vi "DownloadDevMode.vi"(5 "LocalCompiledPath":path, 6 "error in":errorcluster, 9 "Downloader in":refnum<class "Downloader.lvclass">) -> (0 "error out":errorcluster, 2 "Path on Target":path, 3 "Downloader out":refnum<class "Downloader.lvclass">)   [LabVIEW 2014, in "Downloader.lvclass"]
uses:
  Downloader.lvclass
  Downloader.lvclass/Downloader.ctl
  MessageBox/MessageBox.lvclass
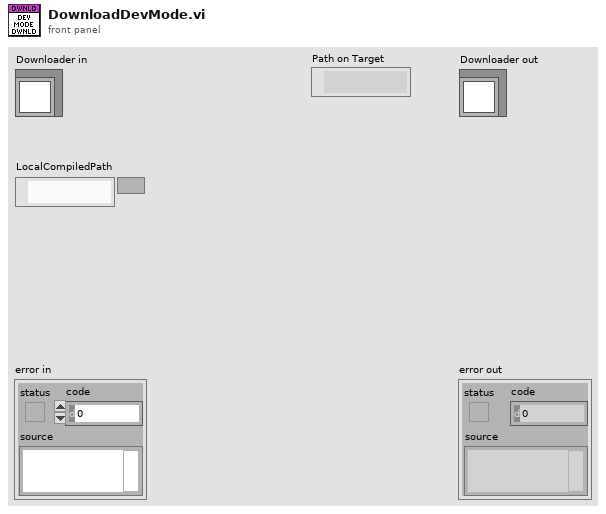
[diagram p1: front panel]
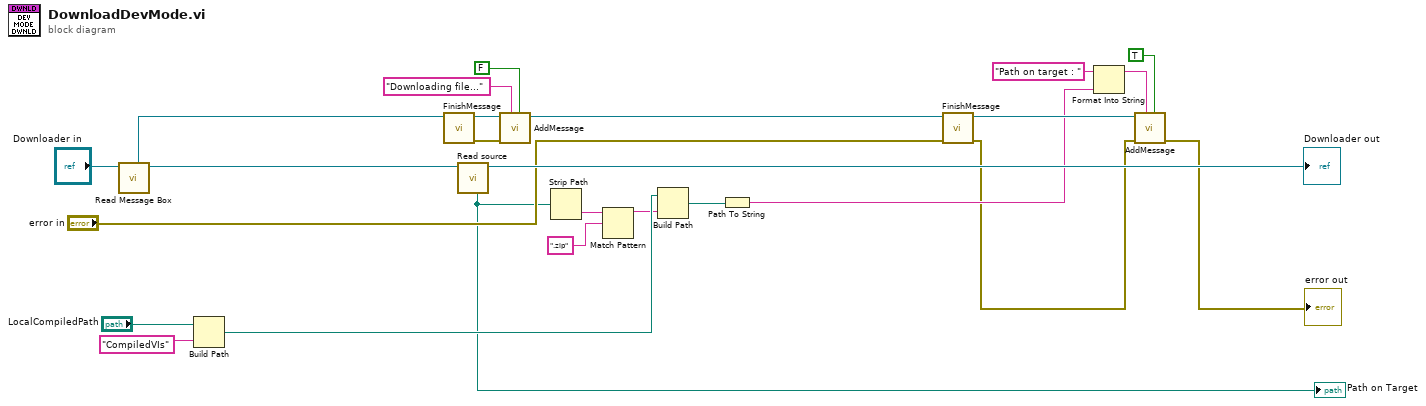
[diagram p0: block diagram]
diagram:
  n1 = call "Read Message Box.vi"("Downloader in"="Downloader in") -> ("Downloader out"=w13:refnum<class "Downloader.lvclass">, "Message Box"=w14:refnum<class "MessageBox.lvclass">)  [unwired: 7 in]
  n2 = Build Path(base path="LocalCompiledPath", name or relative path="CompiledVIs") -> (appended path=w7:path)
  n3 = call "FinishMessage.vi"("MessageBox in"=w14) -> ("error out"=w23:errorcluster, "MessageBox out"=w22:refnum<class "MessageBox.lvclass">)  [unwired: 7 in]
  n4 = call "Read source.vi"("Downloader in"=w13) -> ("Downloader out"=→"Downloader out":refnum<class "Downloader.lvclass">, "source"=w1:path)  [unwired: 7 in]
  "Path on Target" <- w1
  n5 = call "AddMessage.vi"("add newline"=FALSE, "message"="Downloading file...", "error in"=w23, "MessageBox in"=w22) -> ("MessageBox out"=w20:refnum<class "MessageBox.lvclass">)  [unwired: 4 in, 1 out]
  n6 = Strip Path(path=w1) -> (name=w4:string)  [unwired: 1 out]
  n7 = Match Pattern(string=w4, regular expression=".zip") -> (before substring=w2:string)  [unwired: 1 in, 3 out]
  n8 = Build Path(base path=w7, name or relative path=w2) -> (appended path=w5:path)
  n9 = Path To String(path=w5) -> (string=w9:string)
  n10 = call "FinishMessage.vi"("error in"="error in", "MessageBox in"=w20) -> ("error out"=w8:errorcluster, "MessageBox out"=w19:refnum<class "MessageBox.lvclass">)  [unwired: 6 in]
  n11 = Format Into String(initial string="Path on target : ", w9) -> (resulting string=w18:string)  [unwired: 2 in, 1 out]
  n12 = call "AddMessage.vi"("add newline"=TRUE, "message"=w18, "error in"=w8, "MessageBox in"=w19) -> ("error out"=→"error out":errorcluster)  [unwired: 4 in, 1 out]
